vi "Script IO Control.vi"(6 "State":T1={"Worker Library Path"=path "", "Block Label"="", "Types"=[], "Selections"=[], "Icon"={"image type"=0, "image depth"=0, "image"=[], "mask"=[], "colors"=[], "Rectangle"={"left"=0, "top"=0, "right"=0, "bottom"=0}}, "Errors"={"Terminals"=[], "Generate"={"status"=FALSE, "code"=0, "source"=""}, "General"={"status"=FALSE, "code"=0, "source"=""}}, "Calculated Sizes"={"Block Width"=0, "Block Height"=0, "Half Width"=0, "Icon Top"=0, "Icon Bottom"=0, "Label Width"=0, "Half Label"=0, "Label Top"=0, "Text Width"=0, "Half Text"=0, "Text Height"=0, "Label Height"=0, "Expanded Width"=0, "Label Bottom"=0, "Expanded Top"=0, "Expanded Bottom"=0, "Expanded Height"=0, "Min Height"=0, "Max Height"=0}, "Special Terminal Indices"={"Action"=-1, "Init"=-1, "Tag"=-1, "State in"=-1, "State out"=-1, "Error"=-1, "Control"=-1}, "Terminals"=[]}, 8 "error in (no error)":errorcluster, 11 "Refs In":T13) -> (0 "error out":errorcluster, 3 "Refs":T13)   [LabVIEW 2022 SP3, in "FlexBlocks Support.lvlib"]
uses:
  FlexBlocks Support.lvlib
  SM Refs.ctl
  Flex Block/State.ctl
  Type Descriptor.ctl
  Terminal Direction.ctl
  Value Mode.ctl
  Special Terminal.ctl
  <vilib>/picture/picture.llb/imagedata.ctl
  XNode Errors.ctl
  Calculated Sizes.ctl
  Special Terminal Indices.ctl
  Terminal Status.ctl
  Terminal State.ctl
  Terminal Draw Style.ctl
  Flex Block/Flex Block.xnode
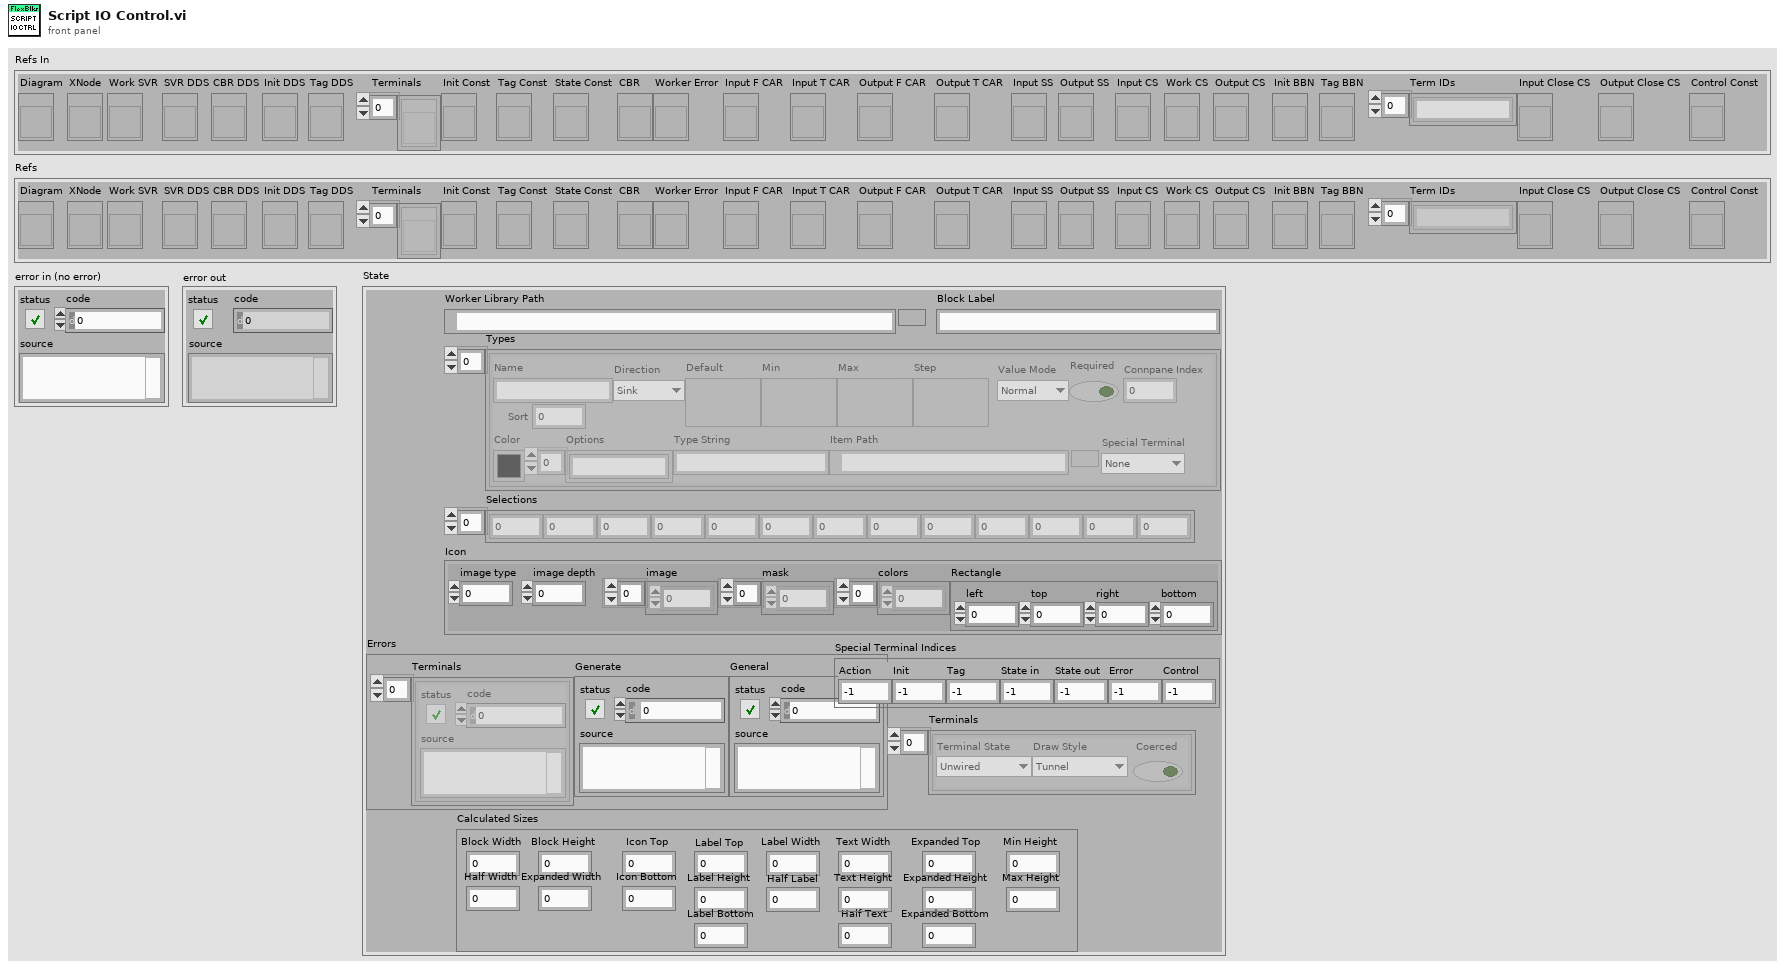
[diagram p1: front panel]
types:
  T1 = typedef "Flex Block.xnode/State.ctl" = cluster{"Worker Library Path":path, "Block Label":string, "Types":T2[], "Selections":i32[], "Icon":T6, "Errors":T7, "Calculated Sizes":T8, "Special Terminal Indices":T9, "Terminals":T10[]}
  T2 = typedef "FlexBlocks Support.lvlib/Type Descriptor.ctl" = cluster{"Name":string, "Direction":T3, "Default":variant, "Min":variant, "Max":variant, "Step":variant, "Value Mode":T4, "Color":u32, "Options":string[], "Type String":string, "Item Path":path, "Required":bool, "Connpane Index":i32, "Special Terminal":T5, "Sort":i32}
  T3 = typedef "FlexBlocks Support.lvlib/Terminal Direction.ctl" = enum16{"Sink", "Source"}
  T4 = typedef "FlexBlocks Support.lvlib/Value Mode.ctl" = enum16{"Normal", "Range", "Select"}
  T5 = typedef "FlexBlocks Support.lvlib/Special Terminal.ctl" = enum16{"None", "Action", "Init", "Tag", "State in", "State out", "Error", "Control"}
  T6 = typedef "imagedata.ctl" = cluster{"image type":i32, "image depth":i32, "image":u8[], "mask":u8[], "colors":u32[], "Rectangle":cluster{"left":i16, "top":i16, "right":i16, "bottom":i16}}
  T7 = typedef "FlexBlocks Support.lvlib/XNode Errors.ctl" = cluster{"Terminals":errorcluster[], "Generate":errorcluster, "General":errorcluster}
  T8 = typedef "FlexBlocks Support.lvlib/Calculated Sizes.ctl" = cluster{"Block Width":i32, "Block Height":i32, "Half Width":i32, "Icon Top":i32, "Icon Bottom":i32, "Label Width":i32, "Half Label":i32, "Label Top":i32, "Text Width":i32, "Half Text":i32, "Text Height":i32, "Label Height":i32, "Expanded Width":i32, "Label Bottom":i32, "Expanded Top":i32, "Expanded Bottom":i32, "Expanded Height":i32, "Min Height":i32, "Max Height":i32}
  T9 = typedef "FlexBlocks Support.lvlib/Special Terminal Indices.ctl" = cluster{"Action":i32, "Init":i32, "Tag":i32, "State in":i32, "State out":i32, "Error":i32, "Control":i32}
  T10 = typedef "FlexBlocks Support.lvlib/Terminal Status.ctl" = cluster{"Terminal State":T11, "Draw Style":T12, "Coerced":bool}
  T11 = typedef "FlexBlocks Support.lvlib/Terminal State.ctl" = enum16{"Unwired", "BadType", "BadRef", "Channel", "Value", "Control Ref"}
  T12 = typedef "FlexBlocks Support.lvlib/Terminal Draw Style.ctl" = enum16{"Tunnel", "BadType", "BadRef", "Channel", "Value", "Control Ref"}
  T13 = typedef "FlexBlocks Support.lvlib/SM Refs.ctl" = cluster{"Diagram":refnum<vi>, "XNode":refnum<vi>, "Work SVR":refnum<vi>, "SVR DDS":refnum<vi>, "CBR DDS":refnum<vi>, "Init DDS":refnum<vi>, "Tag DDS":refnum<vi>, "Terminals":refnum<vi>[], "Init Const":refnum<vi>, "Tag Const":refnum<vi>, "State Const":refnum<vi>, "CBR":refnum<vi>, "Worker Error":refnum<vi>, "Input F CAR":refnum<vi>, "Input T CAR":refnum<vi>, "Output F CAR":refnum<vi>, "Output T CAR":refnum<vi>, "Input SS":refnum<vi>, "Output SS":refnum<vi>, "Input CS":refnum<vi>, "Work CS":refnum<vi>, "Output CS":refnum<vi>, "Init BBN":refnum<vi>, "Tag BBN":refnum<vi>, "Term IDs":string[], "Input Close CS":refnum<vi>, "Output Close CS":refnum<vi>, "Control Const":refnum<vi>}
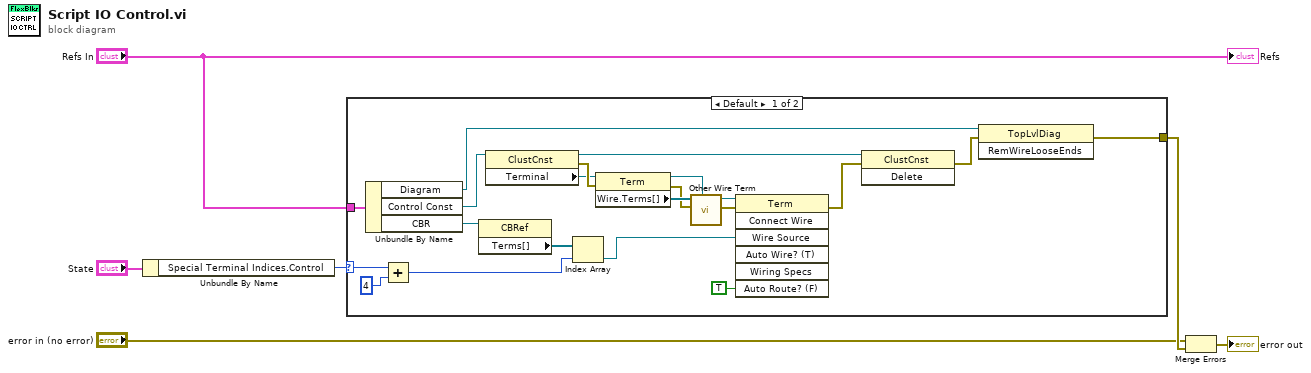
[diagram p0: block diagram]
diagram:
  n1 = Unbundle By Name("State") -> ("Special Terminal Indices.Control"=w5:i32)
  n2 = case shown="Default" w5 {
    selector: w5 -> [w25 _]
    tunnel: "Refs In" -> [w24 _]
    tunnel: [w10 _] -> w3
    frame Default {
      n3 = Unbundle By Name(w24) -> ("Diagram"=w11:refnum<vi>, "Control Const"=w20:refnum<vi>, "CBR"=w23:refnum<vi>)
      n4 = Add(x=w25, y=4) -> (x+y=w21:i32)
      n5 = property class="CBRef"(reference=w23) -> ("Terms[]"=w22:refnum<vi>[])  [unwired: 1 in, 2 out]
      n6 = property class="ClustCnst"(reference=w20) -> (reference out=w15:refnum<vi>, error out=w27:errorcluster, "Terminal"=w19:refnum<vi>)  [unwired: 1 in]
      n7 = Index Array(array=w22, index=w21) -> (element=w13:refnum<vi>)
      n8 = property class="Term"(reference=w19, error in=w27) -> (reference out=w17:refnum<vi>, error out=w16:errorcluster, "Wire.Terms[]"=w18:refnum<vi>[])
      n9 = call "Other Wire Term.vi"("Known Term"=w17, "error in (no error)"=w16, "Wire Terms"=w18) -> ("error out"=w7:errorcluster, "Other Term"=w14:refnum<vi>)  [unwired: 7 in]
      n10 = invoke class="Term" method="Connect Wire"(reference=w14, error in=w7, "Wire Source"=w13, "Auto Route? (F)"=TRUE) -> (error out=w9:errorcluster)  [unwired: 3 in, 6 out]
      n11 = invoke class="ClustCnst" method="Delete"(reference=w15, error in=w9) -> (error out=w8:errorcluster)  [unwired: 1 in, 2 out]
      n12 = invoke class="TopLvlDiag" method="RemWireLooseEnds"(reference=w11, error in=w8) -> (error out=w10:errorcluster)  [unwired: 1 in, 2 out]
    }
    frame -1 {
    }
  }
  n13 = Merge Errors("error in (no error)", w3) -> (→"error out":errorcluster)
  "Refs" <- "Refs In"
